vi "Set All SLSC Switch Properties.vi"(8 "error in (no error)":errorcluster, 10 "SLSC Switch All Properties":T1, 11 "SLSC Sw Custom Device Ref in":T2 format="%.0x") -> (0 "error out":errorcluster, 3 "SLSC Sw Custom Device Ref out":T2 format="%.0x")   [LabVIEW 2017, in "SLSC Switch Scripting.lvlib"]
uses:
  SLSC Switch Scripting.lvlib
  <vilib>/NI Veristand/Custom Device API/Custom Device Item Ref.ctl
  SLSC Switch All Properties.ctl
  <vilib>/NI VeriStand/Custom Device API/Custom Device API.lvlib
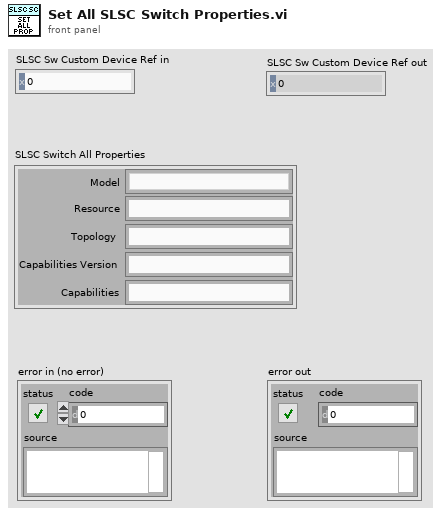
[diagram p1: front panel]
types:
  T1 = typedef "SLSC Switch Scripting.lvlib/SLSC Switch All Properties.ctl" = cluster{"Model":string, "Resource":string, "Topology":string, "Capabilities Version":string, "Capabilities":string}
  T2 = typedef "Custom Device API.lvlib/Custom Device Item Ref.ctl" = u64
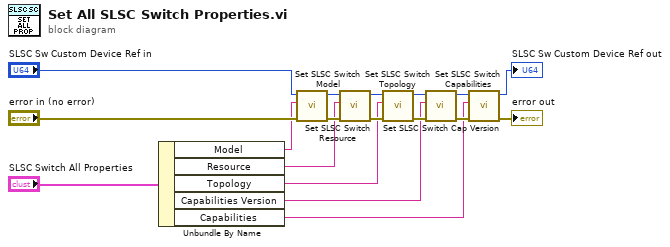
[diagram p0: block diagram]
diagram:
  n1 = Unbundle By Name("SLSC Switch All Properties") -> ("Model"=w1:string, "Resource"=w2:string, "Topology"=w3:string, "Capabilities Version"=w4:string, "Capabilities"=w5:string)
  n2 = call "Set SLSC Switch Model.vi"("error in (no error)"="error in (no error)", "Model"=w1, "SLSC Sw Custom Device Ref in"="SLSC Sw Custom Device Ref in") -> ("error out"=w14:errorcluster, "SLSC Sw Custom Device Ref out"=w12:T2)  [unwired: 7 in]
  n3 = call "Set SLSC Switch Resource.vi"("error in (no error)"=w14, "Resource"=w2, "SLSC Sw Custom Device Ref in"=w12) -> ("error out"=w18:errorcluster, "SLSC Sw Custom Device Ref out"=w17:T2)  [unwired: 7 in]
  n4 = call "Set SLSC Switch Topology.vi"("error in (no error)"=w18, "Topology"=w3, "SLSC Sw Custom Device Ref in"=w17) -> ("error out"=w16:errorcluster, "SLSC Sw Custom Device Ref out"=w15:T2)  [unwired: 7 in]
  n5 = call "Set SLSC Switch Cap Version.vi"("error in (no error)"=w16, "Capabilities Version"=w4, "SLSC Sw Custom Device Ref in"=w15) -> ("error out"=w13:errorcluster, "SLSC Sw Custom Device Ref out"=w10:T2)  [unwired: 7 in]
  n6 = call "Set SLSC Switch Capabilities.vi"("error in (no error)"=w13, "Capabilities"=w5, "SLSC Sw Custom Device Ref in"=w10) -> ("error out"=→"error out":errorcluster, "SLSC Sw Custom Device Ref out"=→"SLSC Sw Custom Device Ref out":T2)  [unwired: 7 in]
